vi "próba.vi"() -> ()   [LabVIEW 2018]
uses:
  <vilib>/sound2/lvsound2.llb/Sampling Mode.ctl
  <vilib>/sound2/lvsound2.llb/Sound Data Format.ctl
  <vilib>/sound2/lvsound2.llb/Sound File Write Open.vi
  <vilib>/sound2/lvsound2.llb/Sound Input Read (DBL).vi
  <vilib>/sound2/lvsound2.llb/Sound File Write (DBL).vi
panel:
  in  "path":path
  in  "stop":bool
  out "Waveform Graph":waveform(dbl)[](graph)
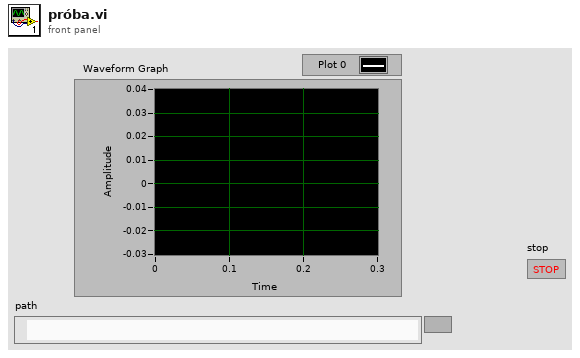
[diagram p1: front panel]
types:
  T1 = typedef "Sound Data Format.ctl" = cluster{"sample rate (S/s)":dbl, "number of channels":i32, "bits per sample":i32}
  T2 = typedef "Sampling Mode.ctl" = i32
  T3 = typedef "Sound Input Task ID.ctl" = u32
  T4 = typedef "Sound File Refnum.ctl" = refnum<file>
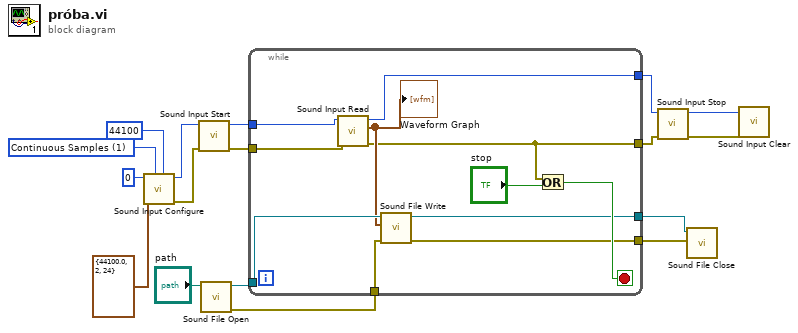
[diagram p0: block diagram]
diagram:
  w16 = T2 1 items=["Finite Samples", "Continuous Samples"] ("sample mode")
  n1 = call <vilib>:"Sound Input Configure.vi"("number of samples/ch"=44100, "sample mode"=w16, "sound format"=T1 {"sample rate (S/s)"=44100.0, "number of channels"=2, "bits per sample"=24}, "device ID"=u32 0) -> ("error out"=w13:errorcluster, "task ID"=w14:T3)  [unwired: 6 in]
  n2 = call <vilib>:"Sound Input Start.vi"("error in (no error)"=w13, "task ID"=w14) -> ("error out"=w11:errorcluster, "task ID out"=w12:T3)  [unwired: 8 in]
  n3 = call-poly <vilib>:"Sound File Open.vi"("path"="path") -> ("error out"=w8:errorcluster, "sound file refnum"=w9:T4)  [unwired: 9 in]
  n4 = while {
    tunnel: w12 -> [w28]
    tunnel: w11 -> [w27]
    tunnel: w9 -> [w26]
    tunnel: w8 -> [w25]
    tunnel: [w23] -> w5
    tunnel: [w21] -> w4
    tunnel: [w19] -> w2
    tunnel: [w18] -> w1
    stop <- w20 stop-if-true
    n5 = call-poly <vilib>:"Sound Input Read.vi"("error in (no error)"=w27, "task ID"=w28) -> ("error out"=w21:errorcluster, "data"=w24:waveform(dbl)[], "task ID out"=w23:T3)  [unwired: 7 in]
    "Waveform Graph" <- w24
    n6 = call-poly <vilib>:"Sound File Write.vi"("error in (no error)"=w25, "data"=w24, "sound file refnum"=w26) -> ("error out"=w18:errorcluster, "sound file refnum out"=w19:T4)  [unwired: 7 in]
    n7 = Or(x=w21, y="stop") -> (x .or. y?=w20:bool)
  }
  n8 = call <vilib>:"Sound Input Stop.vi"("error in (no error)"=w4, "task ID"=w5) -> ("error out"=w6:errorcluster, "task ID out"=w7:T3)  [unwired: 8 in]
  n9 = call <vilib>:"Sound File Close.vi"("error in (no error)"=w1, "sound file refnum"=w2) -> ()  [unwired: 9 in, 1 out]
  n10 = call <vilib>:"Sound Input Clear.vi"("error in (no error)"=w6, "task ID"=w7) -> ()  [unwired: 9 in, 1 out]
